vi "Get Autocal Steps.vi"(0 "VISA Session In":refnum<visa-resource-name>="OXYMAT", 1 "Target Address":u8=16 format="%.0x", 2 "Source Address":u8=208 format="%.0x", 11 "error in (no error)":errorcluster) -> (4 "VISA Session Out":refnum<visa-resource-name>, 6 "Message Header":T2 {"Source Address" format="%.0x"; "Target Address" format="%.0x"}, 10 "Autocal Steps":T1(array[ring]), 13 "Success":bool, 15 "error out":errorcluster)   [LabVIEW 2019, in "Siemens ELAN.lvlib"]
doc: "Using the Siemens ELAN protocol, gets list of Autocal steps (as an array of enumerated values) from the addressed analyzer. Also returns a boolean indicating that the addressed device provided a valid response.\n\n$Revision:: 0 $\n$Modtime:: yy-mm-dd hh:mm $\n$Author:: Dboyd $"
uses:
  Siemens ELAN.lvlib
  Message Header.ctl
  Channel Status.ctl
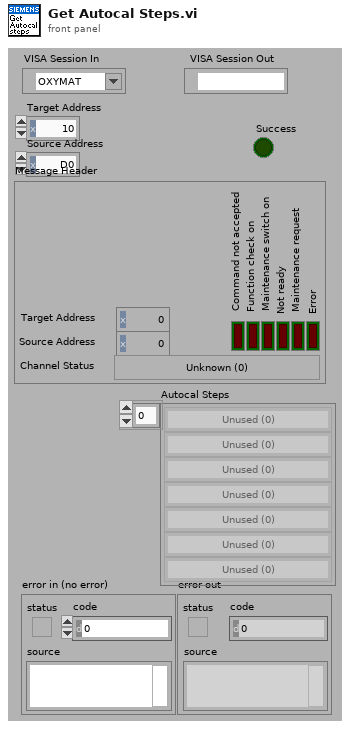
[diagram p1: front panel]
types:
  T1 = enum8{"Unused (0)", "Not Used", "Zero Gas 1", "Zero Gas 2", "Calibration Gas 1", "Calibration Gas 2", "Calibration Gas 3", "Calibration Gas 4", "Sample Gas Purging", "Intermediate Sample Gas Mode", "Signalling Contact", "Unused (>10)"}[]
  T2 = typedef "Siemens ELAN.lvlib/Message Header.ctl" = cluster{"Target Address":u8, "Source Address":u8, "Error":bool, "Maintenance request":bool, "Not ready":bool, "Maintenance switch on":bool, "Function check on":bool, "Command not accepted":bool, "Channel Status":T3}
  T3 = typedef "Siemens ELAN.lvlib/Channel Status.ctl" = enum8{"Unknown (0)", "Warm-up", "Pause", "Standby", "Measure", "Zero calibration", "Adjust component slope", "Unknown (7)", "Adjust curve dip", "Adjust linearization sensitivity", "Adjust temperature compensation", "Adjust pressure compensation", "Adjust linearization zero", "Adjust flow sensor", "Autocal", "Adjust phase", "Zero calibration of O2 sensor", "Synchronous zero calibration", "Purging for synchronous zero calibration", "Adjust analog output", "Adjust analog input", "Cleaning", "Unknown (>21)"}
  T4 = enum8{"Unused (0)", "Not Used", "Zero Gas 1", "Zero Gas 2", "Calibration Gas 1", "Calibration Gas 2", "Calibration Gas 3", "Calibration Gas 4", "Sample Gas Purging", "Intermediate Sample Gas Mode", "Signalling Contact", "Unused (>10)"}
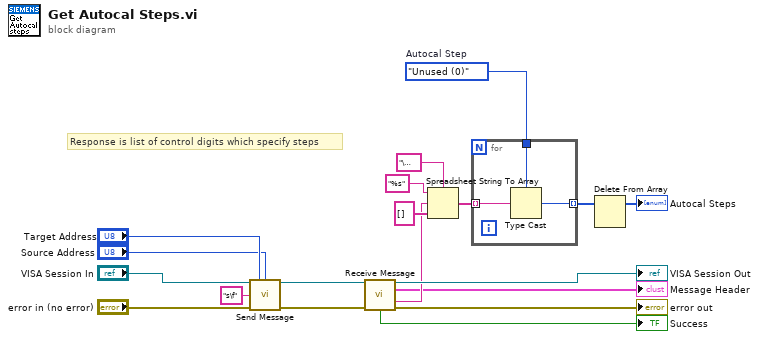
[diagram p0: block diagram]
diagram:
  w3 = T4."Unused (0)"  # Autocal Step
  # "Response is list of control digits which specify steps"
  n1 = call "Send Message.vi"("VISA Session In"="VISA Session In", "Target Address"="Target Address", "Source Address"="Source Address", "Command"="s\f", "error in (no error)"="error in (no error)") -> ("VISA Session Out"=w19:refnum<visa-resource-name>, "error out"=w18:errorcluster)  [unwired: 8 in, 1 out]
  n2 = call "Receive Message.vi"("VISA Session In"=w19, "error in (no error)"=w18) -> ("VISA Session Out"=→"VISA Session Out":refnum<visa-resource-name>, "Message Header"=→"Message Header":T2, "Response"=w9:string, "Success"=→"Success":bool, "error out"=→"error out":errorcluster)  [unwired: 8 in, 1 out]
  n3 = Spreadsheet String To Array(delimiter (Tab)="\u0000", format string="%s", spreadsheet string=w9, array type (2D Dbl)=string[] []) -> (array=w4:string[])
  n4 = for {
    tunnel: w4 -> [w22] mode=indexing
    tunnel: w3 -> [w21]
    tunnel: [w20] -> w2 mode=indexing
    n5 = Type Cast(type=w21, x=w22) -> (*(type *) &x=w20:T4)
  }
  n6 = Delete From Array(array=w2) -> (array with subset deleted=→"Autocal Steps":T1)  [unwired: 2 in, 1 out]
